vi "WPI_AccelerometerAnalogGet.vi"(8 "error in":errorcluster, 11 "AccelerometerDevRef":T2={"DevStatus"={"status"=FALSE, "code"=0, "source"=""}, "Scaling"={"Gain (VoltsPerG)"=0.0, "Center Voltage"=0.0}, "Analog Channels"={"X-Axis"=enum."Invalid", "Y-Axis"=enum."Invalid", "Z-Axis"=enum."Invalid"}, "I2C Bus"=enum."Invalid", "SPI Bus"=enum."Invalid", "Accel Range"=0, "ADXL Axes"={"X-Axis"=FALSE, "Y-Axis"=FALSE, "Z-Axis"=FALSE}, "Handle"=0, "Device Address"=0, "Accel Type"=enum."Analog"} {"Device Address" format="%.0x"; "Accel Range" items=["+/- 2 g", "+/- 4 g", "+/- 8 g", "+/- 16 g"]}) -> (0 "error out":errorcluster, 2 "Accelerations":T1, 3 "AccelerometerDevRef":T2={"DevStatus"={"status"=FALSE, "code"=0, "source"=""}, "Scaling"={"Gain (VoltsPerG)"=0.0, "Center Voltage"=0.0}, "Analog Channels"={"X-Axis"=enum."Invalid", "Y-Axis"=enum."Invalid", "Z-Axis"=enum."Invalid"}, "I2C Bus"=enum."Invalid", "SPI Bus"=enum."Invalid", "Accel Range"=0, "ADXL Axes"={"X-Axis"=FALSE, "Y-Axis"=FALSE, "Z-Axis"=FALSE}, "Handle"=0, "Device Address"=0, "Accel Type"=enum."Analog"} {"Device Address" format="%.0x"; "Accel Range" items=["+/- 2 g", "+/- 4 g", "+/- 8 g", "+/- 16 g"]})   [LabVIEW 2017]
doc: "Returns the current acceleration of the sensor that you specify.\n\nThis software is licensed. Open the labview\\readme\\WPI Robotics Library Open Source License.txt file for more information."
uses:
  <vilib>/Rock Robotics/WPI/Accelerometer/WPI_AccelerometerDevRef.ctl
  <vilib>/Rock Robotics/WPI/Accelerometer/WPI_AccelerometerScaling.ctl
  <vilib>/Rock Robotics/WPI/Accelerometer/WPI_AccelerometerAnalogChannels.ctl
  <vilib>/Rock Robotics/SystemInterfaces/AI/FPGA_AIChannel.ctl
  <vilib>/Rock Robotics/SystemInterfaces/i2clib/i2c_bus.ctl
  <vilib>/Rock Robotics/SystemInterfaces/spilib/spi_bus.ctl
  <vilib>/Rock Robotics/WPI/Accelerometer/ADXL345 Range.ctl
  <vilib>/Rock Robotics/WPI/Accelerometer/WPI_AccelerometerADXL345 Axes.ctl
  <vilib>/Rock Robotics/WPI/AnalogChannel/WPI_AnalogChannelDevRef.ctl
panel:
  # "ADXL"
  # "Analog"
  # "ADXL"
  # "Analog"
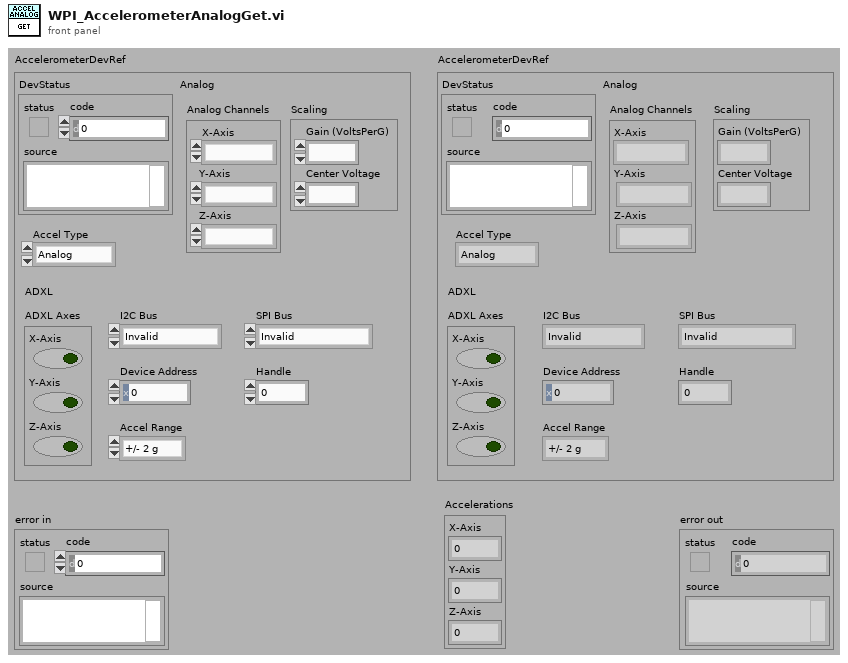
[diagram p1: front panel]
types:
  T1 = cluster{"X-Axis":dbl, "Y-Axis":dbl, "Z-Axis":dbl}
  T2 = typedef "WPI_AccelerometerDevRef.ctl" = cluster{"DevStatus":errorcluster, "Scaling":T3, "Analog Channels":T4, "I2C Bus":T6, "SPI Bus":T7, "Accel Range":T8, "ADXL Axes":T9, "Handle":i32, "Device Address":u8, "Accel Type":enum16{"Analog", "ADXL345 I2C", "ADXL345 SPI", "Internal", "ADXL362 SPI"}}
  T3 = typedef "WPI_AccelerometerScaling.ctl" = cluster{"Gain (VoltsPerG)":dbl, "Center Voltage":dbl}
  T4 = typedef "WPI_AccelerometerAnalogChannels.ctl" = cluster{"X-Axis":T5, "Y-Axis":T5, "Z-Axis":T5}
  T5 = typedef "FPGA_AIChannel.ctl" = enum8{"AI 0", "AI 1", "AI 2", "AI 3", "AI MXP 0", "AI MXP 1", "AI MXP 2", "AI MXP 3", "Invalid"}
  T6 = typedef "i2c_bus.ctl" = enum16{"I2C On-Board", "I2C MXP", "Invalid"}
  T7 = typedef "spi_bus.ctl" = enum16{"SPI On-Board, CS0", "SPI On-Board, CS1", "SPI On-Board, CS2", "SPI On-Board, CS3", "SPI MXP", "Invalid"}
  T8 = typedef "ADXL345 Range.ctl" = u8
  T9 = typedef "WPI_AccelerometerADXL345 Axes.ctl" = cluster{"X-Axis":bool, "Y-Axis":bool, "Z-Axis":bool}
  T10 = typedef "WPI_AnalogChannelDevRef.ctl" = cluster{"DevStatus":errorcluster, "Analog Channel":T5}
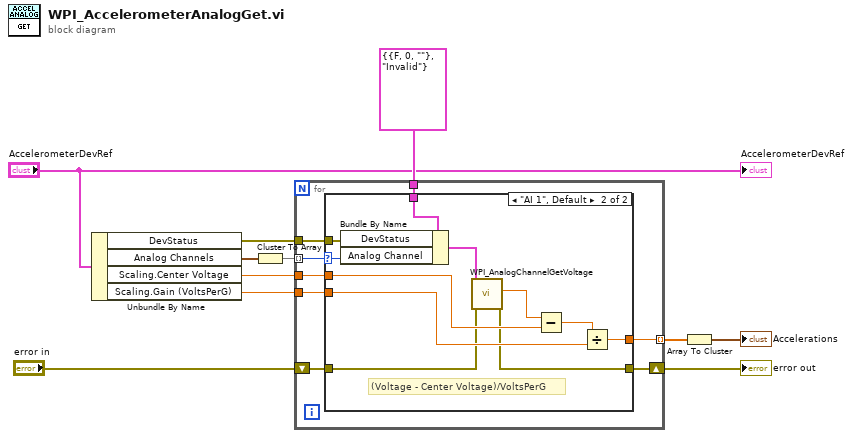
[diagram p0: block diagram]
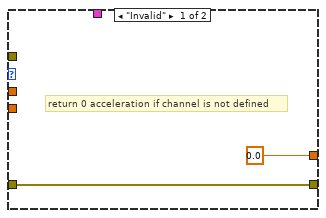
[diagram p2: hidden frame]
diagram:
  n1 = Unbundle By Name("AccelerometerDevRef") -> ("DevStatus"=w6:errorcluster, "Analog Channels"=w9:T4, "Scaling.Center Voltage"=w4:dbl, "Scaling.Gain (VoltsPerG)"=w3:dbl)
  n2 = Cluster To Array(cluster=w9) -> (array=w8:T5[])
  n3 = for {
    shift-right: [w19] -> w11
    shift-left: "error in" -> [w18]
    tunnel: w8 -> [w17] mode=indexing
    tunnel: T10 {"DevStatus"={"status"=FALSE, "code"=0, "source"=""}, "Analog Channel"=enum."Invalid"} ("AIDeviceRef") -> [w16]
    tunnel: w6 -> [w15]
    tunnel: w4 -> [w14]
    tunnel: w3 -> [w13]
    tunnel: [w12] -> w2 mode=indexing
    n4 = case shown="\"AI 1\", Default" w17 {
      selector: w17 -> [_ w31]
      tunnel: [w21 w23] -> w19
      tunnel: w18 -> [w21 w24]
      tunnel: w16 -> [_ w32]
      tunnel: w15 -> [_ w30]
      tunnel: w14 -> [_ w27]
      tunnel: w13 -> [_ w25]
      tunnel: [0.0 ("Voltage") w22] -> w12
      frame "Invalid" {
        # "return 0 acceleration if channel is not defined"
      }
      frame "AI 1", Default {
        # "(Voltage - Center Voltage)/VoltsPerG"
        n5 = Bundle By Name(cluster=w32, "DevStatus"=w30, "Analog Channel"=w31) -> (w29:T10)
        n6 = call <vilib>:"WPI_AnalogChannelGetVoltage.vi"("error in (no error)"=w24, "AIDeviceRef"=w29) -> ("error out"=w23:errorcluster, "Voltage"=w28:dbl)  [unwired: 1 in, 7 out]
        n7 = Subtract(x=w28, y=w27) -> (x-y=w26:dbl)
        n8 = Divide(x=w26, y=w25) -> (x/y=w22:dbl)
      }
    }
  }
  "error out" <- w11
  n9 = Array To Cluster(array=w2) -> (cluster=→"Accelerations":cluster{"[0]":dbl, "[1]":dbl, "[2]":dbl})
  "AccelerometerDevRef" <- "AccelerometerDevRef"
